vi "QueryData.vi"(7 "Message Priority (Normal)":T1=enum."Normal", 8 "error in (no error)":errorcluster, 10 "Start":bool, 11 "Message Enqueuer in":refnum<class "Message Enqueuer.lvclass">) -> (0 "error out":errorcluster)   [LabVIEW 2024, in "4503 Actor.lvlib" / "4503 Actor Msg.lvclass"]
uses:
  4503 Actor Msg.lvclass
  <vilib>/ActorFramework/Message Enqueuer/Message Enqueuer.lvclass
  <vilib>/ActorFramework/Message Enqueuer/Message Priority.ctl
  4503MsgFunc.ctl
  C:/Program Files (x86)/National Instruments/LabVIEW 2024/vi.lib/ActorFramework/Message/Message.lvclass
  4503 Actor Msg.lvclass/4503 Actor Msg.ctl
  <vilib>/ActorFramework/Message Enqueuer/Message Enqueuer.lvclass/Message Enqueuer.ctl
  <vilib>/ActorFramework/Message Priority Queue/Priority Enqueue.vi
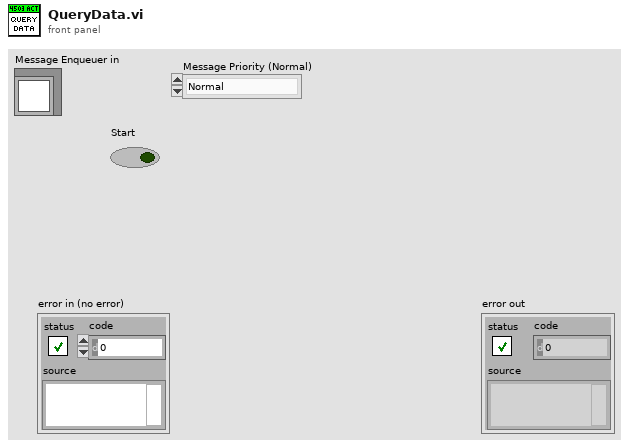
[diagram p1: front panel]
types:
  T1 = typedef "Actor Framework.lvlib/Message Enqueuer.lvclass/Message Priority.ctl" = enum16{"Low", "Normal", "High"}
  T2 = typedef "4503MsgFunc.ctl" = enum16{"StartQuery", "StopQuery", "ZeroAngle", "ClearData"}
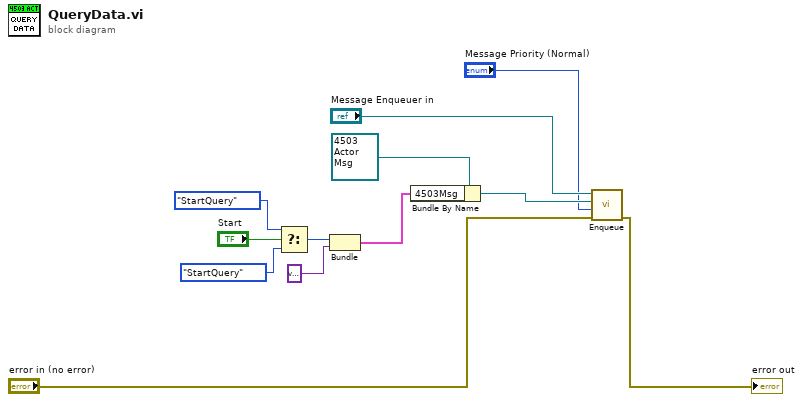
[diagram p0: block diagram]
diagram:
  n1 = Select(t=4503MsgFunc."StartQuery" ("Enum"), s="Start", f=4503MsgFunc."StartQuery" ("Enum")) -> (s? t:f=w7:T2)
  n2 = Bundle("Enum"=w7, variant) -> (w5:cluster{"Enum":T2, variant})  [unwired: 1 in]
  n3 = Bundle By Name(cluster=refnum<class "4503 Actor Msg.lvclass"> refnum ("4503 Actor.lvlib:4503 Actor Msg.lvclass"), "4503Msg"=w5) -> (w4:refnum<class "4503 Actor Msg.lvclass">)
  n4 = call <vilib>:"Enqueue.vi"("error in (no error)"="error in (no error)", "Message Priority (Normal)"="Message Priority (Normal)", "Message"=w4, "Message Enqueuer in"="Message Enqueuer in") -> ("error out"=→"error out":errorcluster)  [unwired: 6 in, 1 out]
